vi "CreateUserEvents.vi"(8 "error in (no error)":errorcluster, 11 "User Event in":refnum<class "User Event.lvclass">) -> (0 "error out":errorcluster, 3 "User Event out":refnum<class "User Event.lvclass">)   [LabVIEW 2016, in "User Event.lvclass"]
uses:
  User Event.lvclass
  TypeDefs/ILCResponse.ctl
  TypeDefs/StopUDPServer.ctl
  User Event.lvclass/User Event.ctl
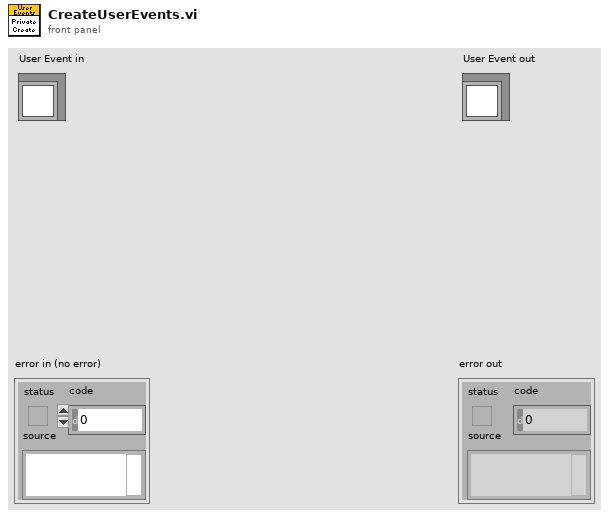
[diagram p1: front panel]
types:
  T1 = typedef "StopUDPServer.ctl" = bool
  T2 = typedef "ILCResponse.ctl" = u8[]
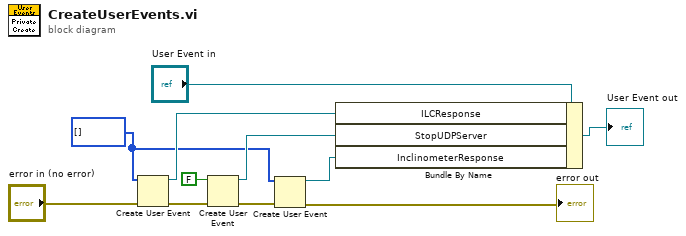
[diagram p0: block diagram]
diagram:
  w4 = T2 [] ("Array")
  n1 = Create User Event(user event datatype=w4, error in="error in (no error)") -> (user event=w10:refnum<user-event>, error out=w5:errorcluster)
  n2 = Create User Event(user event datatype=T1 FALSE ("StopUDPServer"), error in=w5) -> (user event=w6:refnum<user-event>, error out=w3:errorcluster)
  n3 = Create User Event(user event datatype=w4, error in=w3) -> (user event=w1:refnum<user-event>, error out=→"error out":errorcluster)
  n4 = Bundle By Name(cluster="User Event in", "ILCResponse"=w10, "StopUDPServer"=w6, "InclinometerResponse"=w1) -> (→"User Event out":refnum<class "User Event.lvclass">)
